vi "read2002.vi"(8 "error in (no error)":errorcluster, 9 "function (Vdc:1)":u16(ring)=1 items=["ac voltage", "dc voltage", "2-wire resistance", "4-wire resistance", "ac current", "dc current", "frequency", "temperature"]) -> (0 "error out":errorcluster, 1 "medicion":dbl, 2 "Reading Result":string, 3 "Keithley2002 out":refnum<class "Keithley2002.lvclass">)   [LabVIEW 2019, in "Keithley2002.lvclass"]
uses:
  Keithley2002.lvclass
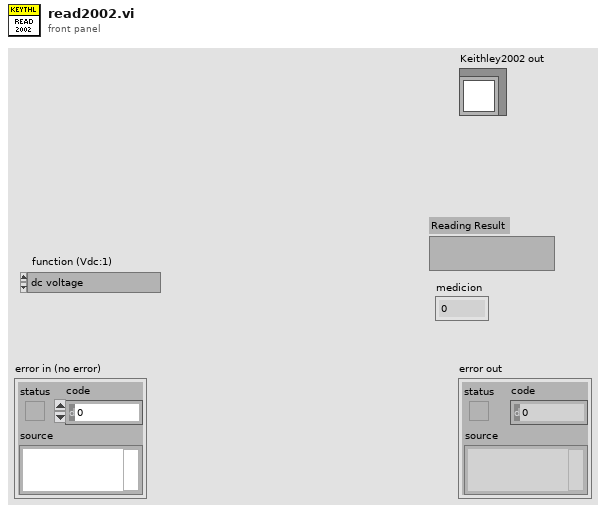
[diagram p1: front panel]
types:
  T1 = cluster{"error":bool, "code":i32, "source":string}
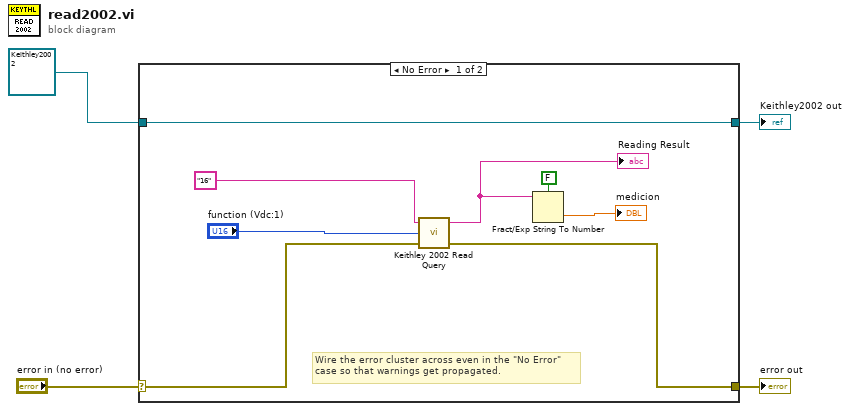
[diagram p0: block diagram]
diagram:
  n1 = case shown="No Error" "error in (no error)" {
    selector: "error in (no error)" -> [w9 w14]
    tunnel: [w8 w14] -> w3
    tunnel: [w12 w13] -> w1
    tunnel: refnum<class "Keithley2002.lvclass"> refnum ("Keithley2002 in") -> [w12 w13]
    frame No Error {
      # "Wire the error cluster across even in the \"No Error\"\ncase so that warnings get propagated."
      n2 = call <instrlib>:"Keithley 2002 Read Query.vi"("error in"=w9, "function (Vdc:1)"="function (Vdc:1)", "GPIB Address"="16") -> ("error out"=w8:T1, "Reading Result"=w7:string)  [unwired: 1 in]
      "Reading Result" <- w7
      n3 = Fract/Exp String To Number(use system decimal point (T)=FALSE, string=w7) -> (number=→"medicion":dbl)  [unwired: 2 in, 1 out]
    }
    frame Error {
    }
  }
  "error out" <- w3
  "Keithley2002 out" <- w1
